vi "NEA_Get Data.vi"(8 "error in (no error)":errorcluster, 10 "Data":T1={"M2 Dataset"={"Read Temp"=273.15, "Feedback"=1, "Set Temp"=273.15}, "M1 Dataset"={"Read Temp"=273.15, "Feedback"=1, "Set Temp"=273.15}, "Comp"=FALSE} {"M1 Dataset"."Set Temp" format="%.1f"; "M1 Dataset"."Feedback" items=["Evap Temp", "Case Temp", "Intec Temp", "TSD  Temp", "Autotune", "Extra"]; "M1 Dataset"."Read Temp" format="%.1f"; "M2 Dataset"."Set Temp" format="%.1f"; "M2 Dataset"."Feedback" items=["Evap Temp", "Case Temp", "Intec Temp", "TSD  Temp", "Autotune", "Extra"]; "M2 Dataset"."Read Temp" format="%.1f"}, 11 "Test in":refnum<class "Test.lvclass">) -> (0 "error out":errorcluster, 3 "Test out":refnum<class "Test.lvclass">)   [LabVIEW 2019, in "Test.lvlib" / "Test.lvclass"]
uses:
  Test.lvclass
  Type Defs/Cobra Data.ctl
  Test.lvclass/Test.ctl
  Test.lvlib
panel:
  # "degC"
  # "degC"
  # "degC"
  # "degC"
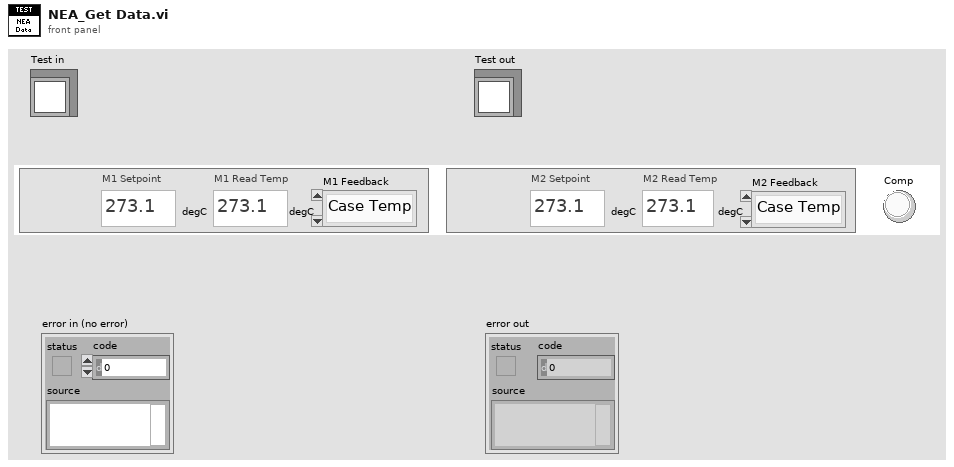
[diagram p1: front panel]
types:
  T1 = typedef "Test.lvlib/Cobra Data.ctl" = cluster{"M2 Dataset":cluster{"Read Temp":dbl, "Feedback":u8, "Set Temp":dbl}, "M1 Dataset":cluster{"Read Temp":dbl, "Feedback":u8, "Set Temp":dbl}, "Comp":bool}
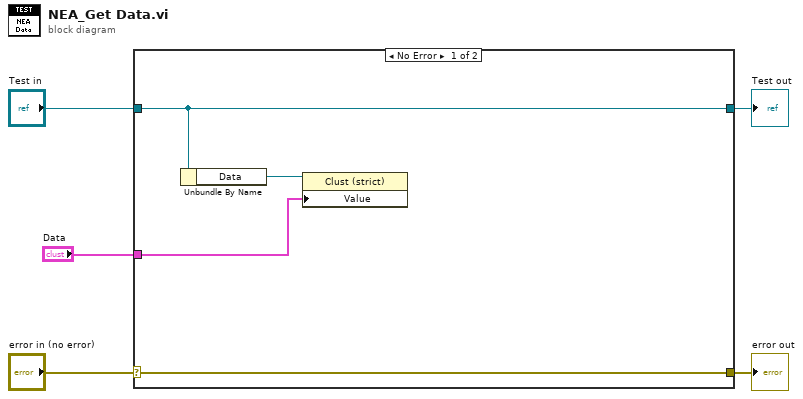
[diagram p0: block diagram]
diagram:
  n1 = case shown="No Error" "error in (no error)" {
    selector: "error in (no error)" -> [w8 w11]
    tunnel: [w8 w11] -> w4
    tunnel: [w9 w10] -> w2
    tunnel: "Test in" -> [w9 w10]
    tunnel: "Data" -> [w6 _]
    frame No Error {
      n2 = Unbundle By Name(w9) -> ("Data"=w7:refnum<vi>)
      n3 = property class="Clust (strict)"(reference=w7, "Value"=w6) -> ()  [unwired: 1 in, 2 out]
    }
    frame Error {
    }
  }
  "error out" <- w4
  "Test out" <- w2
